vi "From Map Array.vi"(0 "Maps":refnum<class "Map.lvclass">[](array[class])) -> (2 "Map":refnum<class "Map.lvclass">)   [LabVIEW 2018, in "Toolkit.lvlib" / "Data.lvlib" / "Map.lvclass"]
uses:
  Map.lvclass
  Map.lvclass/Map.ctl
  Datum/Datum.lvclass
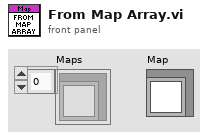
[diagram p1: front panel]
types:
  T1 = cluster{"Key":string, "Value":refnum<class "Datum.lvclass">}[]
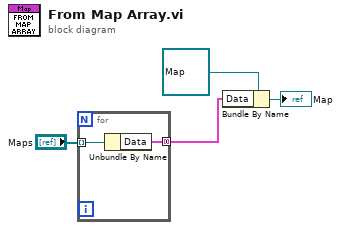
[diagram p0: block diagram]
diagram:
  n1 = for {
    tunnel: "Maps" -> [w6] mode=indexing
    tunnel: [w5] -> w1 mode=concatenating
    n2 = Unbundle By Name(w6) -> ("Data"=w5:T1)
  }
  n3 = Bundle By Name(cluster=refnum<class "Map.lvclass"> refnum ("Toolkit.lvlib:Data.lvlib:Map.lvclass"), "Data"=w1) -> (→"Map":refnum<class "Map.lvclass">)
